vi "ALTS-2015 Read User Details v1.1.vi"(8 "error in (no error)":errorcluster, 11 "User Name":string="Supervisor") -> (0 "error out":errorcluster, 2 "User Info":T1, 3 "User Name Out":string)   [LabVIEW 2013]
doc: "This VI reads the details of the user given in the user name. If the user name is not given then the VI reads the last users details from the registry."
uses:
  <vilib>/Utility/config.llb/NI_LVConfig.lvlib
  SLL VIs/Soliton.lib/File IO/INI/SLL Read a Key of a Section v3.llb/ALTS-2015 SLL Read a Key of a Section for String v3.vi
  Controls/ALTS-2015 User Group Enum2.ctl
  Controls/ALTS-2015 User Info.ctl
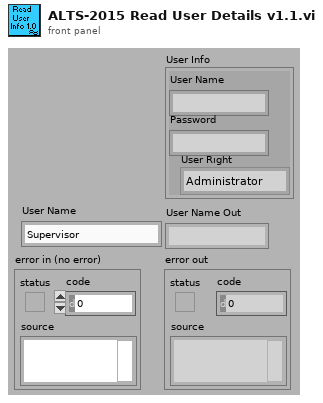
[diagram p1: front panel]
types:
  T1 = typedef "ALTS-2015 User Info.ctl" = cluster{"User Name":string, "Password":string, "User Right":T2}
  T2 = typedef "ALTS-2015 User Group Enum2.ctl" = enum16{"Administrator", "Super User", "Operator"}
  T3 = typedef "NI_LVConfig.lvlib/Config Data RefNum.ctl" = refnum<k1>
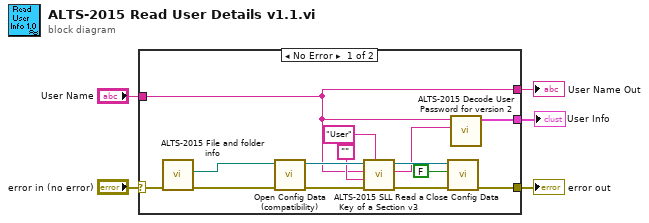
[diagram p0: block diagram]
diagram:
  n1 = case shown="No Error" "error in (no error)" {
    selector: "error in (no error)" -> [w8 w20]
    tunnel: [w13 w20] -> w4
    tunnel: "User Name" -> [w12 _]
    tunnel: [w12 _] -> w2
    tunnel: [w11 _] -> w1
    frame No Error {
      n2 = call "ALTS-2015 File and folder info.vi"("error in (no error)"=w8) -> ("error out"=w7:errorcluster, "INI file path"=w6:path)  [unwired: 5 in, 4 out]
      n3 = call <vilib>:"Open Config Data (compatibility).vi"("error in (no error)"=w7, "configuration file path"=w6) -> ("error out"=w18:errorcluster, "refnum"=w19:T3)  [unwired: 7 in, 1 out]
      n4 = call-poly "ALTS-2015 SLL Read a Key of a Section v3.vi"("Section"="User", "error in (no error)"=w18, "Default Value"="", "Key Name"=w12, "refnum"=w19) -> ("error out"=w16:errorcluster, "Key Value"=w10:string, "refnum out"=w15:T3)  [unwired: 4 in]
      n5 = call <vilib>:"Close Config Data.vi"("error in (no error)"=w16, "write file if changed (T)"=FALSE ("write configuration file? (T)"), "refnum"=w15) -> ("error out"=w13:errorcluster)  [unwired: 7 in, 1 out]
      n6 = call "ALTS-2015 Decode User Password for version 2.vi"("User Value"=w10, "User Name"=w12) -> ("User Info"=w11:T1)  [unwired: 9 in]
    }
    frame Error {
    }
  }
  "error out" <- w4
  "User Name Out" <- w2
  "User Info" <- w1
